vi "Simulated Data.vi"(11 "Polarity":bool) -> (2 "Amplitude Spectrum":T1, 3 "Cluster":T2)   [LabVIEW 2018]
doc: "Generate simulated data."
uses:
  <vilib>/Waveform/WDTOps.llb/WDT Number of Waveform Samples DBL.vi
  <vilib>/measure/madcrms.llb/Basic Averaged DC-RMS for 1 Chan.vi
  <vilib>/measure/NI_MABase.lvlib
  <vilib>/measure/NI_MAPro.lvlib
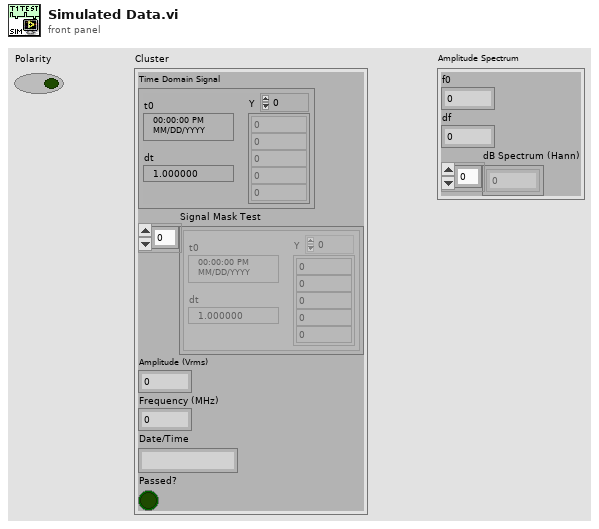
[diagram p1: front panel]
types:
  T1 = cluster{"f0":dbl, "df":dbl, "dB Spectrum (Hann)":dbl[]}
  T2 = cluster{"Time Domain Signal":waveform(dbl), "Signal Mask Test":waveform(dbl)[], "Amplitude (Vrms)":dbl, "Frequency (MHz)":dbl, "Date/Time":string, "Passed?":bool}
  T3 = enum16{"Rectangular (none)", "Hanning", "Low side lobe"}
  T4 = cluster{"waveform out":waveform(dbl), "output values":waveform(dbl)[], "RMS value":dbl, dbl, string, "test passed?":bool}
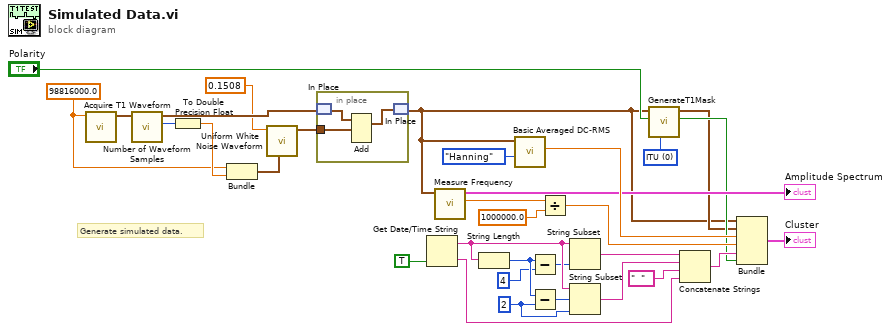
[diagram p0: block diagram]
diagram:
  w6 = 2
  w8 = 98816000.0
  w11 = u16 0 items=["ITU", "EIA/TIA 547-1989"] ("Mask Selector")
  # "Generate simulated data."
  n1 = call "Acquire T1 Waveform.vi"("sampling frequency"=w8) -> ("Waveform"=w21:waveform(dbl))  [unwired: 9 in, 1 out]
  n2 = call-poly <vilib>:"Number of Waveform Samples.vi"("waveform in"=w21) -> ("number of samples"=w24:i32, "waveform out"=w22:waveform(dbl))  [unwired: 8 in, 1 out]
  n3 = To Double Precision Float(number=w24) -> (double precision float=w26:dbl)
  n4 = Bundle(w8, w26) -> (w25:cluster{dbl, dbl})  [unwired: 1 in]
  n5 = call <vilib>:"Uniform White Noise Waveform.vi"("sampling info"=w25, "amplitude"=0.1508) -> ("signal out"=w23:waveform(dbl))  [unwired: 8 in, 1 out]
  n6 = in-place {
    in-place-border: w23 -> [w35]
    n7 = in-place-match #1(w22) -> (w34:waveform(dbl))
    n8 = Add ("Add Waveforms.vi")(1:w35, 2:w34) -> (0:w33:waveform(dbl))  [unwired: 1 in, 1 out]
    n9 = in-place-match #1(w33) -> (w5:waveform(dbl))
  }
  n10 = Get Date/Time String(want seconds? (F)=TRUE) -> (date string=w31:string, time string=w32:string)  [unwired: 2 in]
  n11 = call "Measure Frequency.vi"("Waveform"=w5) -> ("frequency"=w20:dbl, "exported spectrum (dB)"=→"Amplitude Spectrum":T1)  [unwired: 7 in, 2 out]
  n12 = String Length(string=w31) -> (length=w28:i32)
  n13 = call-poly <vilib>:"Basic Averaged DC-RMS.vi"("window"=T3."Hanning", "signal in"=w5) -> ("RMS value"=w16:dbl)  [unwired: 6 in, 3 out]
  n14 = Subtract(x=w28, y=4) -> (x-y=w29:i32)
  n15 = Subtract(x=w28, y=w6) -> (x-y=w30:i32)
  n16 = Divide(x=w20, y=1000000.0) -> (x/y=w17:dbl)
  n17 = String Subset(string=w31, length (rest)=w29) -> (substring=w2:string)  [unwired: 1 in]
  n18 = String Subset(string=w31, offset (0)=w30, length (rest)=w6) -> (substring=w1:string)
  n19 = call "GenerateT1Mask.vi"("Mask Selector"=w11, "Polarity"="Polarity", "Waveform"=w5) -> ("test passed?"=w13:bool, "output values"=w12:waveform(dbl)[])  [unwired: 6 in, 1 out]
  n20 = Concatenate Strings(w2, w1, "  ", w32) -> (w18:string)
  n21 = Bundle("waveform out"=w5, "output values"=w12, "RMS value"=w16, w17, w18, "test passed?"=w13) -> (→"Cluster":T4)  [unwired: 1 in]
